vi "New Test.vi"(8 "error in (no error)":errorcluster, 10 "NewTest":T1(array[cluster]), 11 "TestBench in":refnum<class "TestBench.lvclass">) -> (0 "error out":errorcluster, 3 "TestBench out":refnum<class "TestBench.lvclass">)   [LabVIEW 2019, in "TestBench.lvlib" / "TestBench.lvclass"]
uses:
  TestBench.lvclass
  TestBench.lvclass/TestBench.ctl
  UnitTestEngine/UnitTestEngine Messages/NewTest Msg/NewTest Msg.lvclass/NewTest Msg.ctl
  <vilib>/ActorFramework/Message Enqueuer/Message Enqueuer.lvclass/Message Enqueuer.ctl
  <vilib>/ActorFramework/Message Enqueuer/Enqueue.vi
  UnitTestEngine/UnitTestEngine Messages/NewTest Msg/NewTest Msg.lvclass
  C:/Program Files (x86)/National Instruments/LabVIEW 2019/vi.lib/ActorFramework/Message/Message.lvclass
  <vilib>/ActorFramework/Message Priority Queue/Priority Enqueue.vi
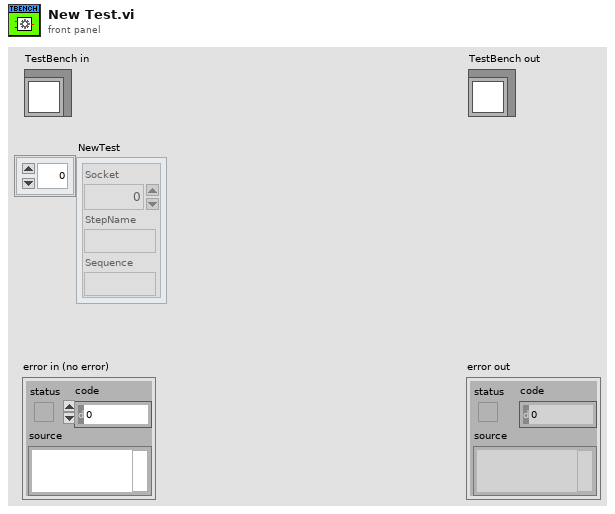
[diagram p1: front panel]
types:
  T1 = cluster{"Socket":i32, "StepName":string, "Sequence":string}[]
  T2 = map{string, refnum<class "Message Enqueuer.lvclass">}
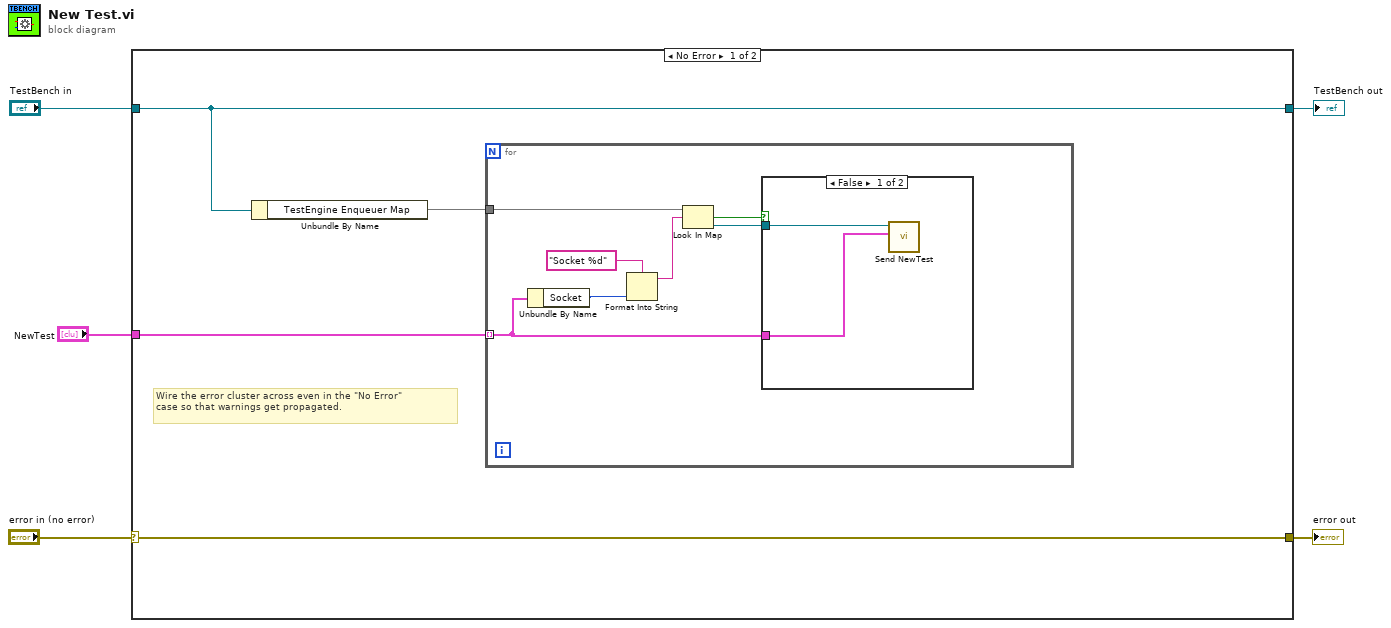
[diagram p0: block diagram]
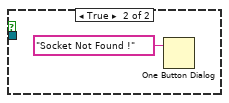
[diagram p2: hidden frame]
diagram:
  n1 = case shown="No Error" "error in (no error)" {
    selector: "error in (no error)" -> [w9 w21]
    tunnel: [w9 w21] -> w4
    tunnel: [w8 w20] -> w2
    tunnel: "TestBench in" -> [w8 w20]
    tunnel: "NewTest" -> [w7 _]
    frame No Error {
      # "Wire the error cluster across even in the \"No Error\"\ncase so that warnings get propagated."
      n2 = Unbundle By Name(w8) -> ("TestEngine Enqueuer Map"=w6:T2)
      n3 = for {
        tunnel: w7 -> [w13] mode=indexing
        tunnel: w6 -> [w16]
        n4 = Unbundle By Name(w13) -> ("Socket"=w11:i32)
        n5 = Format Into String(format string="Socket %d", w11) -> (resulting string=w10:string)  [unwired: 2 in, 1 out]
        n6 = Look In Map(map=w16, key=w10) -> (key not found?=w14:bool, value=w15:refnum<class "Message Enqueuer.lvclass">)  [unwired: 1 in]
        n7 = case shown="False" w14 {
          tunnel: w15 -> [w18 _]
          tunnel: w13 -> [w17 _]
          frame False {
            n8 = call "Send NewTest.vi"("NewTest"=w17, "Message Enqueuer"=w18) -> ()  [unwired: 8 in, 2 out]
          }
          frame True {
            n9 = One Button Dialog(message="Socket Not Found !") -> ()  [unwired: 1 in, 1 out]
          }
        }
      }
    }
    frame Error {
    }
  }
  "error out" <- w4
  "TestBench out" <- w2
